vi "FFTBoost.vi"(5 "PhaseCorrection":dbl[](array[numeric]), 7 "CompensationCoefficients":dbl[](array[numeric])=[1.0, 1.0, 0.0, 0.0, 0.0], 10 "mutedData":dbl[](array[numeric])=array[1605632 elements]) -> (2 "boostedData":dbl[](array[numeric]))   [LabVIEW 2016]
uses:
  <vilib>/Analysis/2dsp.llb/Real FFT.vi
  <vilib>/Analysis/2dsp.llb/Inverse Real FFT.vi
  <vilib>/Analysis/NI_AALPro.lvlib
panel:
  out "CallCount":dbl
  out "Waveform Graph":cluster{i32, i32, dbl[]}[](graph)
  # "NOTE- This VI DOES NOT preserve means- they should be calculated before, and re-added after, compensation"
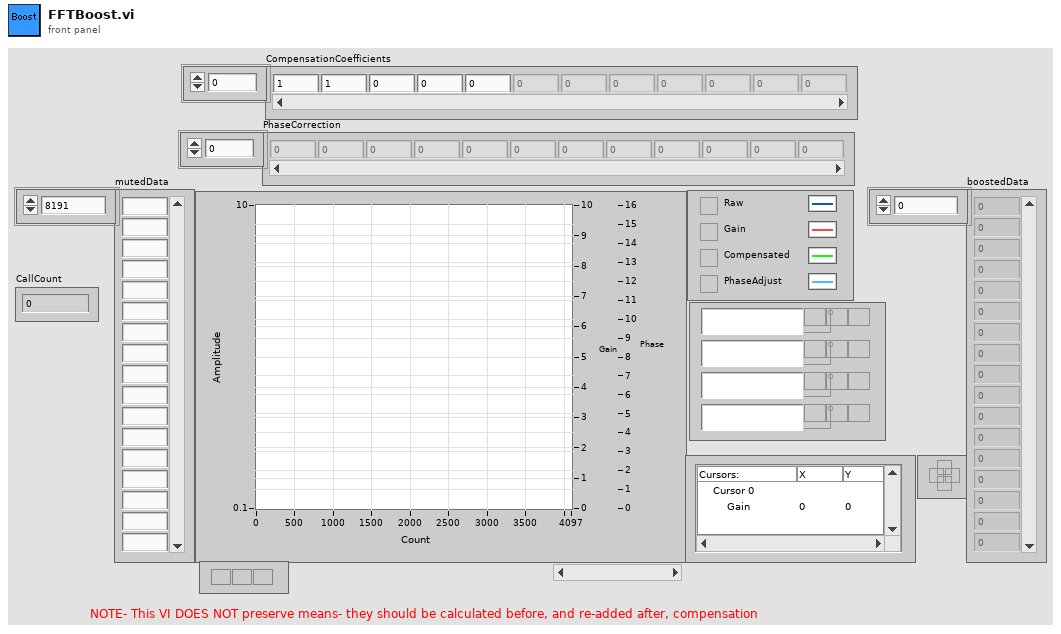
[diagram p1: front panel]
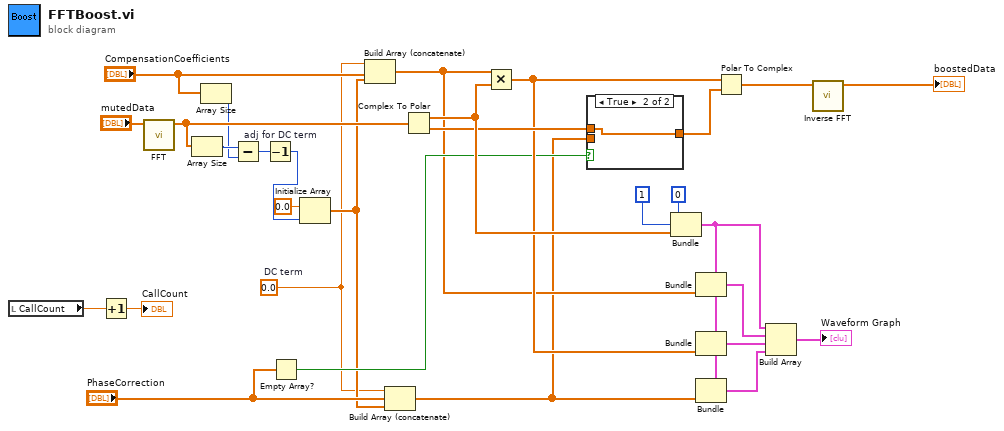
[diagram p0: block diagram]
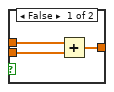
[diagram p2: hidden frame]
diagram:
  w2 = 0.0  # DC term
  n1 = local read "CallCount"() -> (w24:dbl)
  n2 = Increment(x=w24) -> (x+1=→"CallCount":dbl)
  n3 = call-poly <vilib>:"FFT.vi"("X"="mutedData") -> ("FFT {X}"=w12:cdb[])  [unwired: 2 in, 8 out]
  n4 = Array Size(array=w12) -> (size(s)=w11:i32)
  n5 = Array Size(array="CompensationCoefficients") -> (size(s)=w10:i32)
  n6 = Subtract(x=w11, y=w10) -> (x-y=w9:i32)
  n7 = Decrement "adj for DC term"(x=w9) -> (x-1=w3:i32)
  n8 = Empty Array?(array="PhaseCorrection") -> (empty?=w17:bool)
  n9 = Initialize Array(0.0 ("element"), w3) -> (w4:dbl[])
  n10 = Build Array (concatenate)(w2, "CompensationCoefficients", w4) -> (w8:dbl[])
  n11 = Build Array (concatenate)(w2, "PhaseCorrection", w4) -> (w5:dbl[])
  n12 = Complex To Polar(r * e^(i*theta)=w12) -> (r=w22:dbl[], theta=w21:dbl[])
  n13 = Multiply(x=w8, y=w22) -> (x*y=w19:dbl[])
  n14 = case shown="True" w17 {
    tunnel: w5 -> [w30 _]
    tunnel: w21 -> [w31 w33]
    tunnel: [w32 w33] -> w20
    frame False {
      n15 = Add(x=w31, y=w30) -> (x+y=w32:dbl[])
    }
    frame True {
    }
  }
  n16 = Bundle(0, 1, w22) -> (w15:cluster{i32, i32, dbl[]})  [unwired: 1 in]
  n17 = Bundle(cluster=w15, w8) -> (w28:cluster{i32, i32, dbl[]})  [unwired: 2 in]
  n18 = Bundle(cluster=w15, w19) -> (w27:cluster{i32, i32, dbl[]})  [unwired: 2 in]
  n19 = Bundle(cluster=w15, w5) -> (w14:cluster{i32, i32, dbl[]})  [unwired: 2 in]
  n20 = Polar To Complex(1:w20, 2:w19) -> (0:w18:cdb[])
  n21 = Build Array(w15, w28, w27, w14) -> (→"Waveform Graph":cluster{i32, i32, dbl[]}[])
  n22 = call-poly <vilib>:"Inverse FFT.vi"("FFT {X}"=w18) -> ("X"=→"boostedData":dbl[])  [unwired: 1 in, 9 out]
